vi "Read Enable.vi"(8 "error in (no error)":errorcluster, 11 "JsonReportPlugin in":refnum<class "JsonReportPlugin.lvclass">) -> (0 "error out":errorcluster, 2 "Enable":bool, 3 "JsonReportPlugin out":refnum<class "JsonReportPlugin.lvclass">)   [LabVIEW 2015, in "JsonReportPlugin.lvclass"]
uses:
  JsonReportPlugin.lvclass
  JsonReportPlugin.lvclass/JsonReportPlugin.ctl
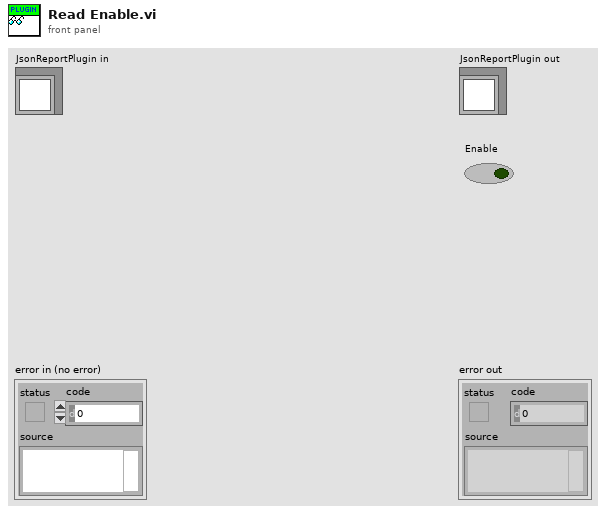
[diagram p1: front panel]
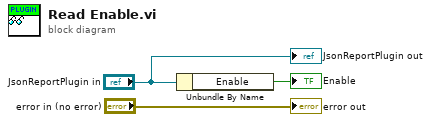
[diagram p0: block diagram]
diagram:
  n1 = Unbundle By Name("JsonReportPlugin in") -> ("Enable"=→"Enable":bool)
  "error out" <- "error in (no error)"
  "JsonReportPlugin out" <- "JsonReportPlugin in"
